vi "Add Digital Pattern.vi"(8 "error in (no error)":errorcluster, 10 "Page Data in":T1 {"Node Ptr" format="%.0x"}, 11 "State queue in":string[](array[string])) -> (0 "error out":errorcluster, 2 "Page Data out":T1 {"Node Ptr" format="%.0x"}, 3 "State queue out":string[](array[string]))   [LabVIEW 2015, in "Engine Simulation Toolkit System Explorer.lvlib"]
uses:
  Engine Simulation Toolkit System Explorer.lvlib
  Digital Patterns Page Data.ctl
  <vilib>/NI Veristand/Custom Device API/Custom Device Item Ref.ctl
  Digital Pattern.ctl
  Digital Pattern Base.ctl
  Digital Pattern Remove Edge.ctl
  Digital Pattern Add Pulse.ctl
  <vilib>/NI Veristand/Custom Device API/Custom Device Channel Type.ctl
  Shared/Constants and GUIDs.vi
  Shared/Properties.vi
  <vilib>/NI Veristand/Custom Device API/Set Item Property (String).vi
  <vilib>/NI Veristand/Custom Device API/Custom Device API.lvlib
  Shared/Engine Simulation Toolkit Shared.lvlib
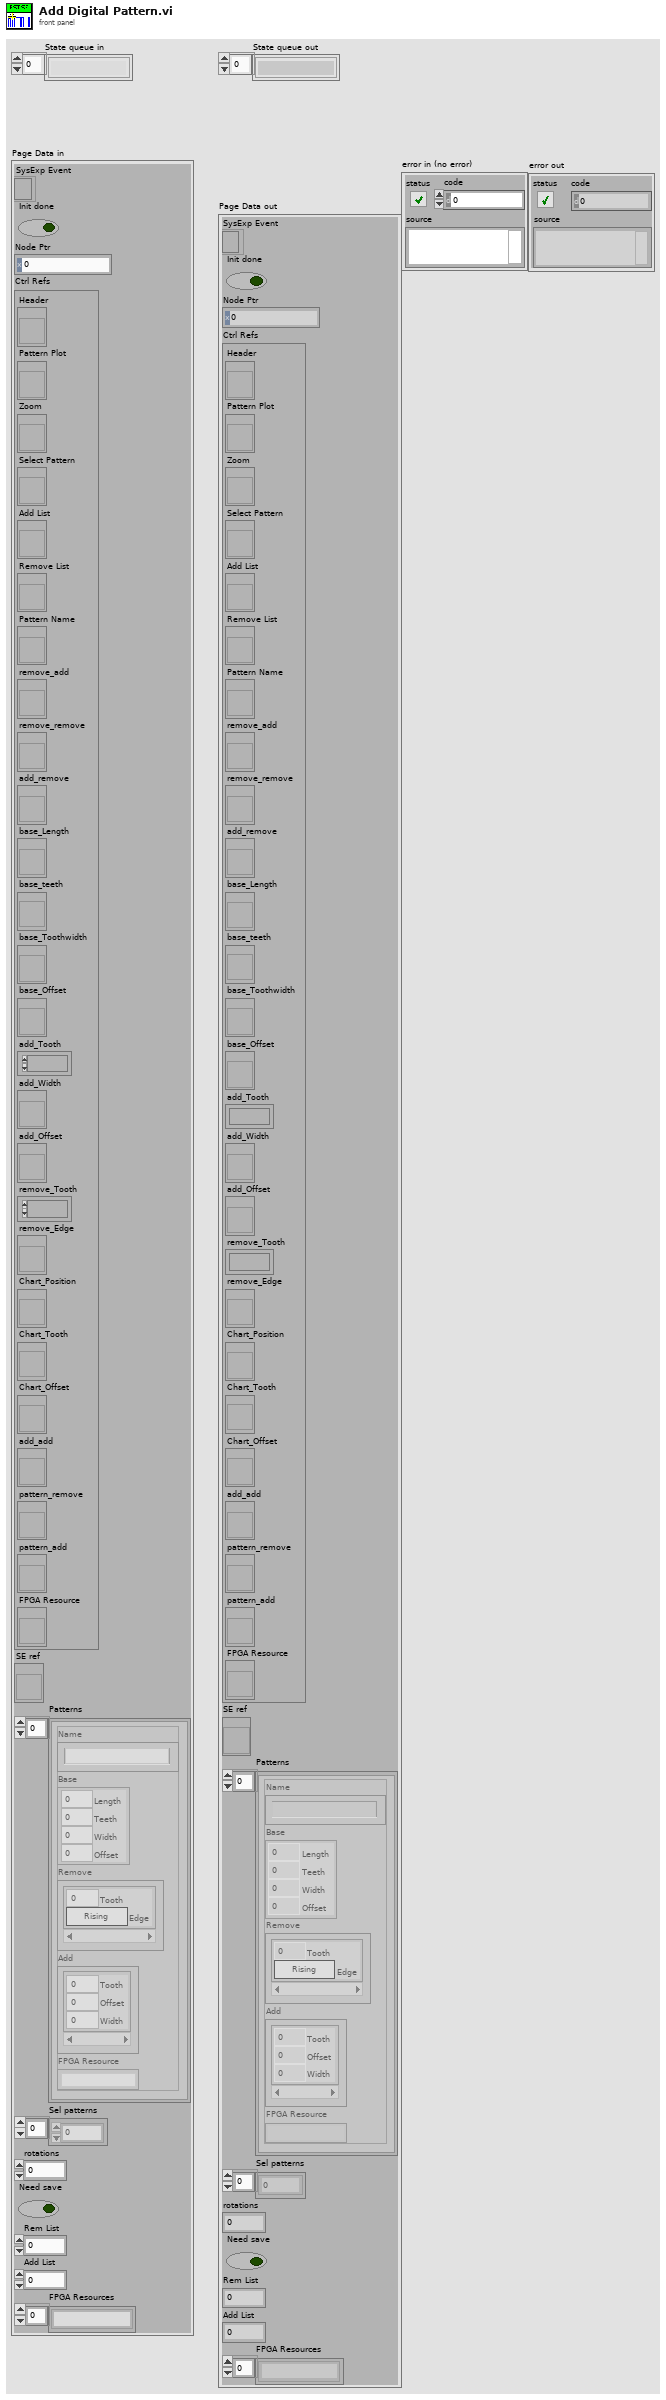
[diagram p1: front panel]
types:
  T1 = typedef "Engine Simulation Toolkit System Explorer.lvlib/Digital Patterns Page Data.ctl" = cluster{"SysExp Event":refnum<event-registration>, "Init done":bool, "Node Ptr":T2, "Ctrl Refs":cluster{"Header":refnum<vi>, "Pattern Plot":refnum<vi>, "Zoom":refnum<vi>, "Select Pattern":refnum<vi>, "Add List":refnum<vi>, "Remove List":refnum<vi>, "Pattern Name":refnum<vi>, "remove_add":refnum<vi>, "remove_remove":refnum<vi>, "add_remove":refnum<vi>, "base_Length":refnum<vi>, "base_teeth":refnum<vi>, "base_Toothwidth":refnum<vi>, "base_Offset":refnum<vi>, "add_Tooth":refnum<vi>, "add_Width":refnum<vi>, "add_Offset":refnum<vi>, "remove_Tooth":refnum<vi>, "remove_Edge":refnum<vi>, "Chart_Position":refnum<vi>, "Chart_Tooth":refnum<vi>, "Chart_Offset":refnum<vi>, "add_add":refnum<vi>, "pattern_remove":refnum<vi>, "pattern_add":refnum<vi>, "FPGA Resource":refnum<vi>}, "SE ref":refnum<vi>, "Patterns":T3[], "Sel patterns":i32[], "rotations":u16, "Need save":bool, "Rem List":i32, "Add List":i32, "FPGA Resources":string[]}
  T2 = typedef "Custom Device API.lvlib/Custom Device Item Ref.ctl" = u64
  T3 = typedef "Engine Simulation Toolkit System Explorer.lvlib/Digital Pattern.ctl" = cluster{"Name":string, "Base":T4, "Remove":T5[], "Add":T6[], "FPGA Resource":string}
  T4 = typedef "Engine Simulation Toolkit System Explorer.lvlib/Digital Pattern Base.ctl" = cluster{"Length":dbl, "Teeth":u16, "Width":dbl, "Offset":dbl}
  T5 = typedef "Engine Simulation Toolkit System Explorer.lvlib/Digital Pattern Remove Edge.ctl" = cluster{"Tooth":u16, "Edge":bool}
  T6 = typedef "Engine Simulation Toolkit System Explorer.lvlib/Digital Pattern Add Pulse.ctl" = cluster{"Tooth":u16, "Offset":dbl, "Width":dbl}
  T7 = typedef "Custom Device API.lvlib/Custom Device Channel Type.ctl" = enum16{"Input", "Output"}
  T8 = typedef "Engine Simulation Toolkit Shared.lvlib/Bitfile EST Version.ctl" = enum16{"1.0", "1.1", "1.2", "1.3"}
  T9 = typedef "Engine Simulation Toolkit Shared.lvlib/Channel.ctl" = cluster{"Name":string, "Units":string, "Default":dbl, "Description":string}
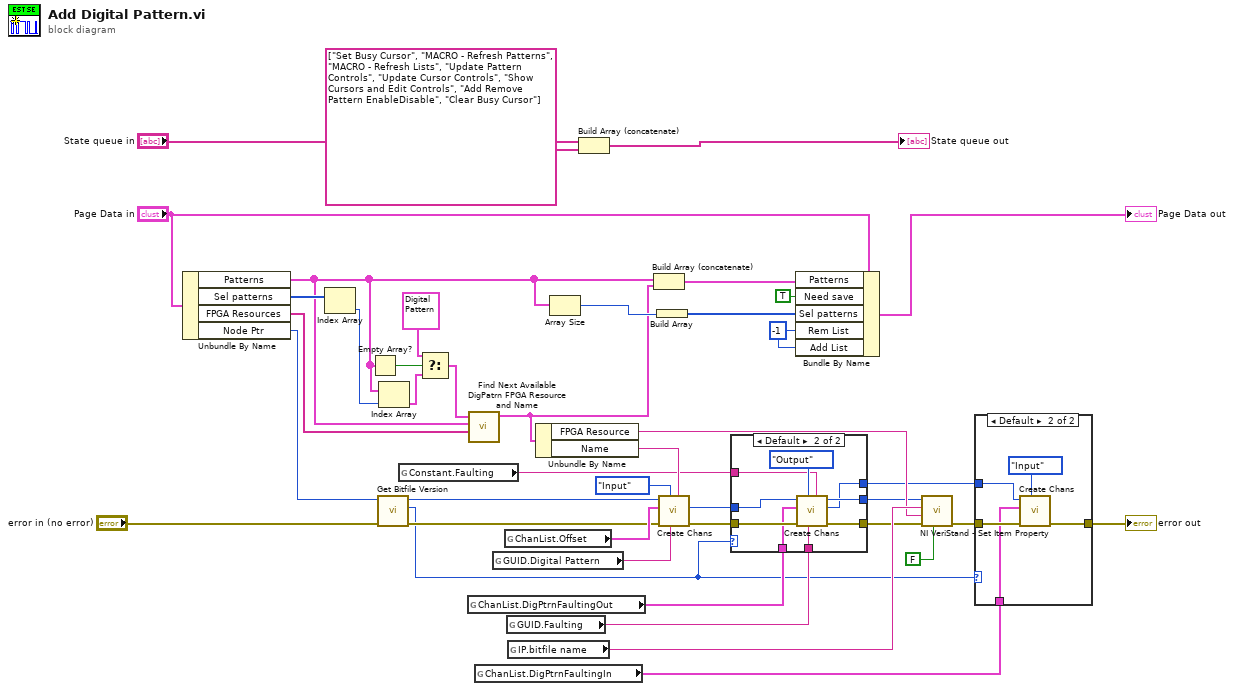
[diagram p0: block diagram]
diagram:
  w41 = -1 ("Rem List")
  n1 = Unbundle By Name("Page Data in") -> ("Patterns"=w27:T3[], "Sel patterns"=w36:i32[], "FPGA Resources"=w28:string[], "Node Ptr"=w4:T2)
  n2 = Index Array(array=w36) -> (element=w38:i32)  [unwired: 1 in]
  n3 = Empty Array?(array=w27) -> (empty?=w25:bool)
  n4 = call "Get Bitfile Version.vi"("error in (no error)"="error in (no error)", "Item Ref in"=w4) -> ("error out"=w5:errorcluster, "EST version enum"=w2:T8, "Item Ref out"=w3:T2)  [unwired: 6 in, 1 out]
  n5 = Index Array(array=w27, index=w38) -> (element=w35:T3)
  n6 = global read "Constants and GUIDs.vi" "Constant.Faulting"() -> (w1:string)
  n7 = Select(t=T3 {"Name"="New Pattern", "Base"={"Length"=360.0, "Teeth"=60, "Width"=1.0, "Offset"=-0.5}, "Remove"=[{"Tooth"=58, "Edge"=FALSE}, {"Tooth"=59, "Edge"=FALSE}], "Add"=[], "FPGA Resource"=""} ("s? t:f"), s=w25, f=w35) -> (s? t:f=w26:T3)
  n8 = global read "Constants and GUIDs.vi" "ChanList.DigPtrnFaultingOut"() -> (w11:T9[])
  n9 = call "Find Next Available DigPatrn FPGA Resource and Name.vi"("FPGA Resources"=w28, "Patterns"=w27, "New Pattern in"=w26) -> ("New Pattern out"=w24:T3)  [unwired: 8 in]
  n10 = global read "Constants and GUIDs.vi" "ChanList.DigPtrnFaultingIn"() -> (w8:T9[])
  n11 = global read "Constants and GUIDs.vi" "GUID.Digital Pattern"() -> (w19:string)
  n12 = global read "Constants and GUIDs.vi" "ChanList.Offset"() -> (w20:T9[])
  n13 = global read "Constants and GUIDs.vi" "GUID.Faulting"() -> (w6:string)
  n14 = global read "Properties.vi" "IP.bitfile name"() -> (w17:string)
  n15 = Unbundle By Name(w24) -> ("FPGA Resource"=w16:string, "Name"=w22:string)
  n16 = Array Size(array=w27) -> (size(s)=w42:i32)
  n17 = Build Array (concatenate)("State queue in", string[] ["Set Busy Cursor", "MACRO - Refresh Patterns", "MACRO - Refresh Lists", "Update Pattern Controls", "Update Cursor Controls", "Show Cursors and Edit Controls", "Add Remove Pattern EnableDisable", "Clear Busy Cursor"]) -> (→"State queue out":string[])
  n18 = Build Array (concatenate)(w27, w24) -> (w37:T3[])
  n19 = Build Array(w42) -> (w39:i32[])
  n20 = call "Create Chans.vi"("New Section Name (none)"=w22, "new section GUID (\"\":del prot)"=w19, "Type"=Custom_Device_Channel_Type."Input", "error in (no error)"=w5, "Channels"=w20, "Section Ptr"=w3) -> ("error out"=w18:errorcluster, "new section ref"=w13:T2)  [unwired: 2 in, 2 out]
  n21 = case shown="Default" w2 {
    tunnel: w18 -> [w43 w53]
    tunnel: [w43 w52] -> w14
    tunnel: w13 -> [w44 w51]
    tunnel: [w44 w50] -> w12
    tunnel: w11 -> [_ w49]
    tunnel: [_ w47] -> w9
    tunnel: w6 -> [_ w46]
    tunnel: w1 -> [_ w45]
    frame "1.0".."1.2" {
    }
    frame Default {
      n22 = call "Create Chans.vi"("New Section Name (none)"=w45, "new section GUID (\"\":del prot)"=w46, "Type"=Custom_Device_Channel_Type."Output", "error in (no error)"=w53, "Channels"=w49, "Section Ptr"=w51) -> ("error out"=w52:errorcluster, "new section ref"=w47:T2, "Section Ptr dup"=w50:T2)  [unwired: 2 in, 1 out]
    }
  }
  n23 = Bundle By Name(cluster="Page Data in", "Patterns"=w37, "Need save"=TRUE, "Sel patterns"=w39, "Rem List"=w41, "Add List"=w41) -> (→"Page Data out":T1)
  n24 = call-poly <vilib>:"NI VeriStand - Set Item Property.vi"("Binary String (T)"=FALSE, "error in (no error)"=w14, "Value"=w16, "Property Name"=w17, "Item Ref in"=w12) -> ("error out"=w10:errorcluster)  [unwired: 4 in, 2 out]
  n25 = case shown="Default" w2 {
    tunnel: w10 -> [w54 w59]
    tunnel: w9 -> [_ w58]
    tunnel: w8 -> [_ w57]
    tunnel: [w54 w55] -> w7
    frame "1.0".."1.2" {
    }
    frame Default {
      n26 = call "Create Chans.vi"("Type"=Custom_Device_Channel_Type."Input", "error in (no error)"=w59, "Channels"=w57, "Section Ptr"=w58) -> ("error out"=w55:errorcluster)  [unwired: 4 in, 3 out]
    }
  }
  "error out" <- w7
